vi "State Colors.vi"(8 "error in (no error)":errorcluster, 11 "Sequence Config in":refnum<class "Sequence Config.lvclass">) -> (0 "error out":errorcluster, 2 "State Colors":map{string, string}(c390), 3 "Sequence Config out":refnum<class "Sequence Config.lvclass">)   [LabVIEW 2020, in "VolatusSeqConfig.lvlib" / "Sequence Config.lvclass"]
uses:
  Sequence Config.lvclass
  Sequence Config.lvclass/Sequence Config.ctl
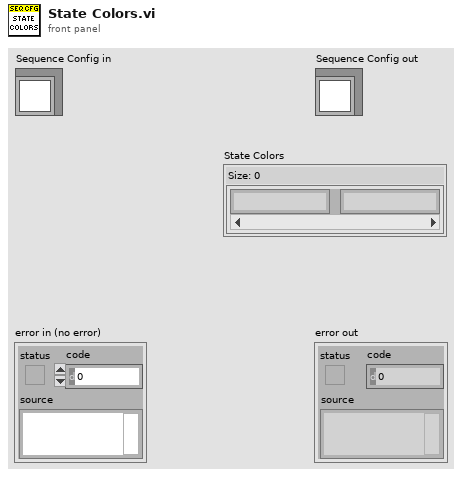
[diagram p1: front panel]
types:
  T1 = typedef "VolatusSeqConfig.lvlib/State.ctl" = cluster{"Name":string, "Steps":T2[], "Transitions":refnum<class "Transition Config.lvclass">[], "Comment":string, "Color":string}
  T2 = typedef "VolatusSeqConfig.lvlib/Step.ctl" = cluster{"Time":dbl, "Commands":refnum<class "Command Config.lvclass">[]}
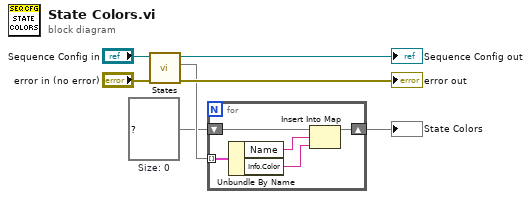
[diagram p0: block diagram]
diagram:
  w2 = map{string, string} {}  # Size: 0
  n1 = call "States.vi"("error in (no error)"="error in (no error)", "Sequence Config in"="Sequence Config in") -> ("error out"=→"error out":errorcluster, "States"=w3:map{string, T1}, "Sequence Config out"=→"Sequence Config out":refnum<class "Sequence Config.lvclass">)  [unwired: 7 in]
  n2 = for {
    tunnel: w3 -> [w12] mode=indexing
    shift-right: [w8] -> w1
    shift-left: w2 -> [w11]
    n3 = Unbundle By Name(w12) -> ("Name"=w10:string, "Info.Color"=w9:string)
    n4 = Insert Into Map(map in=w11, key=w10, value=w9) -> (map out=w8:map{string, string})  [unwired: 2 out]
  }
  "State Colors" <- w1
